vi "lectura-escritura.vi"() -> ()   [LabVIEW 2016]
panel:
  in  "Stop Button":bool
  out "String 2":string
  in  "String":string
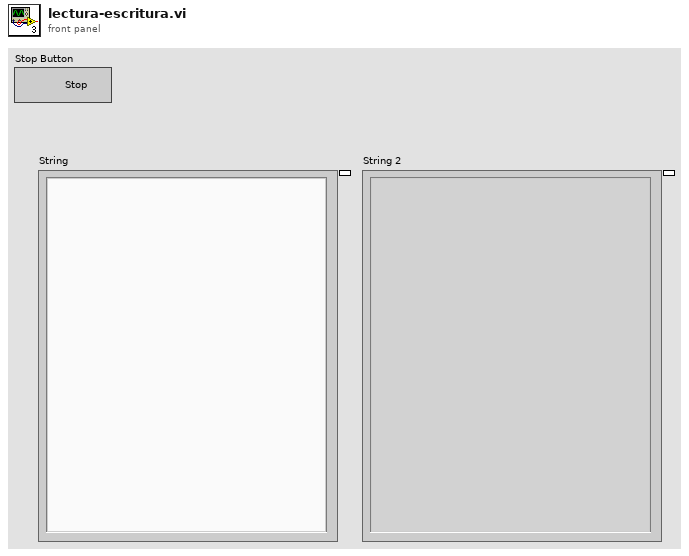
[diagram p1: front panel]
types:
  T1 = enum16{"Read", "Write", "ReadWrite", "BufferedRead", "BufferedReadWrite"}
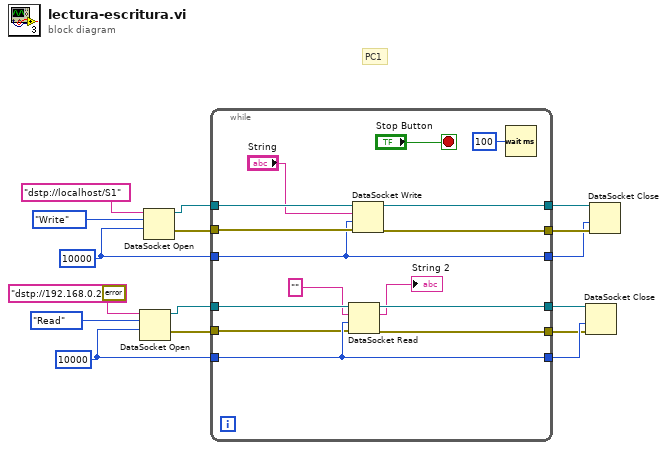
[diagram p0: block diagram]
diagram:
  w7 = 10000 ("ms timeout (10000)")
  w10 = 10000 ("ms timeout (10000)")
  (unwired) errorcluster {"status"=FALSE, "code"=0, "source"=""} ("error constant")
  # "PC1"
  n1 = DataSocket Open(9:w7, 10:T1."Read" ("mode"), 11:"dstp://192.168.0.2/S2" ("URL")) -> (0:w4:errorcluster, 3:w1:refnum<k13>)  [unwired: 1 in]
  n2 = DataSocket Open(9:w10, 10:T1."Write" ("mode"), 11:"dstp://localhost/S1" ("URL")) -> (0:w13:errorcluster, 3:w16:refnum<k13>)  [unwired: 1 in]
  n3 = while {
    tunnel: w16 -> [w29]
    tunnel: [w28] -> w15
    tunnel: [w27] -> w14
    tunnel: w13 -> [w26]
    tunnel: w10 -> [w25]
    tunnel: [w25] -> w9
    tunnel: w1 -> [w20]
    tunnel: [w21] -> w2
    tunnel: [w22] -> w3
    tunnel: w4 -> [w23]
    tunnel: w7 -> [w24]
    tunnel: [w24] -> w8
    stop <- "Stop Button" stop-if-true
    n4 = DataSocket Read(8:w23, 9:w24, 10:"", 11:w20) -> (0:w22:errorcluster, 2:→"String 2":string, 3:w21:refnum<k13>)  [unwired: 1 in, 4 out]
    n5 = DataSocket Write(8:w26, 9:w25, 10:"String", 11:w29) -> (0:w27:errorcluster, 3:w28:refnum<k13>)  [unwired: 1 out]
    n6 = Wait (ms)(milliseconds to wait=u32 100) -> ()  [unwired: 1 out]
  }
  n7 = DataSocket Close(8:w3, 9:w8, 11:w2) -> ()  [unwired: 2 out]
  n8 = DataSocket Close(8:w14, 9:w9, 11:w15) -> ()  [unwired: 2 out]
